vi "CANOpen_Initialize RT Driver.vi"(8 "error in (no error)":errorcluster, 11 "Device Reference in":T24 format="%.0x") -> (0 "error out":errorcluster, 3 "Configuration Cluster":T10={"Driver Settings"={"CANOpen Bus Settings"={"CANOpen Interface Name"=0, "Baud Rate"=0, "Termination"=FALSE, "Sync Period (ms)"=10, "Enable 9881"=FALSE, "RIO Device"=0, "Enable SYNC"=FALSE, "Scan & Print"=FALSE}, "Nodes"=[], "Node Ids"=[]}, "Data References"={"Hardware Input"={"FIFO"=refnum, "Channel Pairs"={"Chan Refs"=[], "Prev. Values"=[]}}, "Hardware Output"={"FIFO"=refnum, "Channel Pairs"={"Block Refs"=[], "Prev. Values"=[]}}}, "Bus Commands"={"Hardware Output"={"FIFO"=refnum, "Channel Pairs"={"Chan Refs"=[], "Prev. Values"=[]}}, "Hardware Input"={"FIFO"=refnum}}, "SDO Asynch"={"List SDO"={"FIFO Req"=refnum, "Req Chan."={"Chan Refs"=[], "NodeIndex"=[]}, "FIFO Resp"=refnum, "Resp Chan."={"Chan Refs"=[]}, "Node IDs"=[], "FIFO array"=[]}, "HW Dyn Write"={"FIFO Req"=refnum, "FIFO Resp"=refnum, "Req Chan."={"Chan Refs"=[], "Node IDs"=[]}, "Resp Chan."={"Chan Refs"=[]}}, "HW Dyn Read"={"FIFO Req"=refnum, "FIFO Resp"=refnum, "Req Chan."={"Chan Refs"=[], "Node IDs"=[]}, "Resp Chan."={"Chan Refs"=[]}}}, "Status NMT"={"Hardware Output"={"FIFO"=refnum, "Channel Pairs"={"Chan Refs"=[], "Prev. Values"=[], "Node index"=[]}}, "Hardware Input"={"FIFO"=refnum, "Channel Pairs"={"Chan Refs"=[], "Prev. Values"=[], "Node index"=[]}}}} {"Status NMT"."Hardware Output"."Channel Pairs"."Chan Refs"."Data Reference" format="%.0x"; "Status NMT"."Hardware Input"."Channel Pairs"."Chan Refs" format="%.0x"; "SDO Asynch"."HW Dyn Read"."Resp Chan."."Chan Refs" format="%.0x"; "SDO Asynch"."HW Dyn Read"."Req Chan."."Chan Refs" format="%.0x"; "SDO Asynch"."HW Dyn Write"."Resp Chan."."Chan Refs" format="%.0x"; "SDO Asynch"."HW Dyn Write"."Req Chan."."Chan Refs" format="%.0x"; "SDO Asynch"."List SDO"."Resp Chan."."Chan Refs" format="%.0x"; "SDO Asynch"."List SDO"."Req Chan."."Chan Refs" format="%.0x"; "Bus Commands"."Hardware Output"."Channel Pairs"."Chan Refs" format="%.0x"; "Data References"."Hardware Input"."Channel Pairs"."Chan Refs" format="%.0x"; "Data References"."Hardware Output"."Channel Pairs"."Block Refs"."Data Reference" format="%.0x"; "Driver Settings"."CANOpen Bus Settings"."Baud Rate" items=["1 Mbit/s"=0, "800 kbit/s"=1, "500 kbit/s"=2, "250 kbit/s"=3, "125 kbit/s"=4, "50 kbit/s"=6, "20 kbit/s"=7, "10 kbit/s"=8]; "Driver Settings"."CANOpen Bus Settings"."CANOpen Interface Name" items=["CANopen01", "CANopen02", "CANopen03", "CANopen04", "CANopen05", "CANopen06", "CANopen07", "CANopen08", "CANopen09", "CANopen10", "CANopen11", "CANopen12", "CANopen13", "CANopen14", "CANopen15", "CANopen16", "CANopen17", "CANopen18", "CANopen19", "CANopen20", "CANopen21", "CANopen22", "CANopen23", "CANopen24", "CANopen25", "CANopen26", "CANopen27", "CANopen28", "CANopen29", "CANopen30", "CANopen31", "CANopen32"]; "Driver Settings"."Nodes"."NMT"."Node init static SDO state" items=["start remote node"=1, "enter pre-operational"=128]; "Driver Settings"."Nodes"."NMT"."Node run state" items=["start remote node"=1, "stop remote node"=2, "enter pre-operational"=128, "reset node"=129, "reset communication"=130]; "Driver Settings"."Nodes"."Dynamic SDOs"."Block Data" format="%.0x"; "Driver Settings"."Nodes"."RPDOs"."PDO Channel" items=["PDO 1", "PDO 2", "PDO 3", "PDO 4"]; "Driver Settings"."Nodes"."TPDOs"."PDO Channel" items=["PDO 1", "PDO 2", "PDO 3", "PDO 4"]; "Driver Settings"."Nodes"."SDOs"."Block Data" format="%.0x"})   [LabVIEW 2013]
uses:
  <vilib>/NI Veristand/Custom Device API/Custom Device Item Ref.ctl
  CANOpen_Settings.ctl
  CANOpen_Node Settings.ctl
  Shared Code/CANOpen_Bus Settings.ctl
  Shared Code/CANOpen Interface Name.ctl
  <vilib>/CANopenLib/CANOPEN.llb/CANopen BaudRate.ctl
  CANOpen_Node Message Settings.ctl
  Shared Code/CANOpen_PDO Settings.ctl
  Shared Code/CANOpen_PDO Parameter Settings.ctl
  Shared Code/CANOpen_PDO Data Type.ctl
  System Explorer/SubVIs/CANopen Byte Order.ctl
  Shared Code/CANOpen_SDO Settings.ctl
  CANOpen_NMT Settings.ctl
  Async VIs/CANOpen_Main/SubVIs/CanOpen_NMT_Config.ctl
  Async VIs/CANOpen_Main/SubVIs/CanOpen_NMT_Static detect.ctl
  Async VIs/CANOpen_Main/SubVIs/CanOpen_Main Node Ids.ctl
  CANOpen_VS Data Refs.ctl
  <vilib>/NI Veristand/Custom Device API/Data Reference.ctl
  <vilib>/NI Veristand/Custom Device API/Block Data Reference.ctl
  CANOpen_VS Bidirectional Data Refs.ctl
  CANOpen_VS SDOs Data Refs.ctl
  Async VIs/CANOpen_Main/SubVIs/CanOpen_SDO Dynamic queue.ctl
  Shared Code/CANOpen_SDO queue W data.ctl
  Shared Code/CANOpen_SDO queue mode.ctl
  Shared Code/CANOpen_PDO Data Type in queue.ctl
  CANOpen_VS Status Management Data Refs.ctl
  Async VIs/CANOpen_Main/SubVIs/CanOpen_NMT_HWOut_ChannelPairs.ctl
  Async VIs/CANOpen_Main/SubVIs/CanOpen_NMT_HWIn_ChannelPairs.ctl
  CANOpen_xPDO VS Refs.ctl
  Shared Code/CANOpen_Get PDO Channel from Name.vi
  Shared Code/CANOpen_SetGet PDO Parameter Settings.vi
  CANOpen_SetGet NMT Settings.vi
  CANOpen_Initialize VS BiDirectional Data Refs.vi
  CANOpen_Search Channel Ref.vi
  CANOpen_Search Channel Refs.vi
  CANOpen_Initialize VS NMT Data Refs.vi
  <vilib>/NI Veristand/Custom Device Tools/Custom Device Utility Library/NI VeriStand - Search for All Items by GUID.vi
  <vilib>/NI Veristand/Custom Device API/Get Item Property (Variant).vi
  Shared Code/CANOpen Addon GUID Lookup Global.vi
  <vilib>/NI Veristand/Custom Device API/NI VeriStand - Get Item Children.vi
  <vilib>/NI Veristand/Custom Device Tools/Custom Device Utility Library/NI VeriStand - Search for Item by GUID.vi
  <vilib>/NI Veristand/Custom Device API/NI VeriStand - Get Channel Data Reference.vi
  <vilib>/NI Veristand/Custom Device API/NI VeriStand - Get Channel Block Data References.vi
  <vilib>/NI Veristand/Custom Device Tools/Custom Device Utility Library/Custom Device Utility Library.lvlib
  CANOpen Addon Custom Device.lvlib
  <vilib>/NI Veristand/Custom Device API/Custom Device API.lvlib
  Debug/SubVIs/Global debug.vi
panel:
  out "Array":T1[](array[typedef]) {"NMT"."Node init static SDO state" items=["start remote node"=1, "enter pre-operational"=128]; "NMT"."Node run state" items=["start remote node"=1, "stop remote node"=2, "enter pre-operational"=128, "reset node"=129, "reset communication"=130]; "Dynamic SDOs"."Block Data" format="%.0x"; "RPDOs"."PDO Channel" items=["PDO 1", "PDO 2", "PDO 3", "PDO 4"]; "RPDOs"."Parameters"."Bit Offset" max=8 step=1; "RPDOs"."Parameters"."Byte Offset" max=8 step=1; "TPDOs"."PDO Channel" items=["PDO 1", "PDO 2", "PDO 3", "PDO 4"]; "TPDOs"."Parameters"."Bit Offset" max=8 step=1; "TPDOs"."Parameters"."Byte Offset" max=8 step=1; "SDOs"."Block Data" format="%.0x"}
  # "LSB"
  # "MSB"
  # "LSB"
  # "MSB"
  # "LSB"
  # "MSB"
  # "LSB"
  # "MSB"
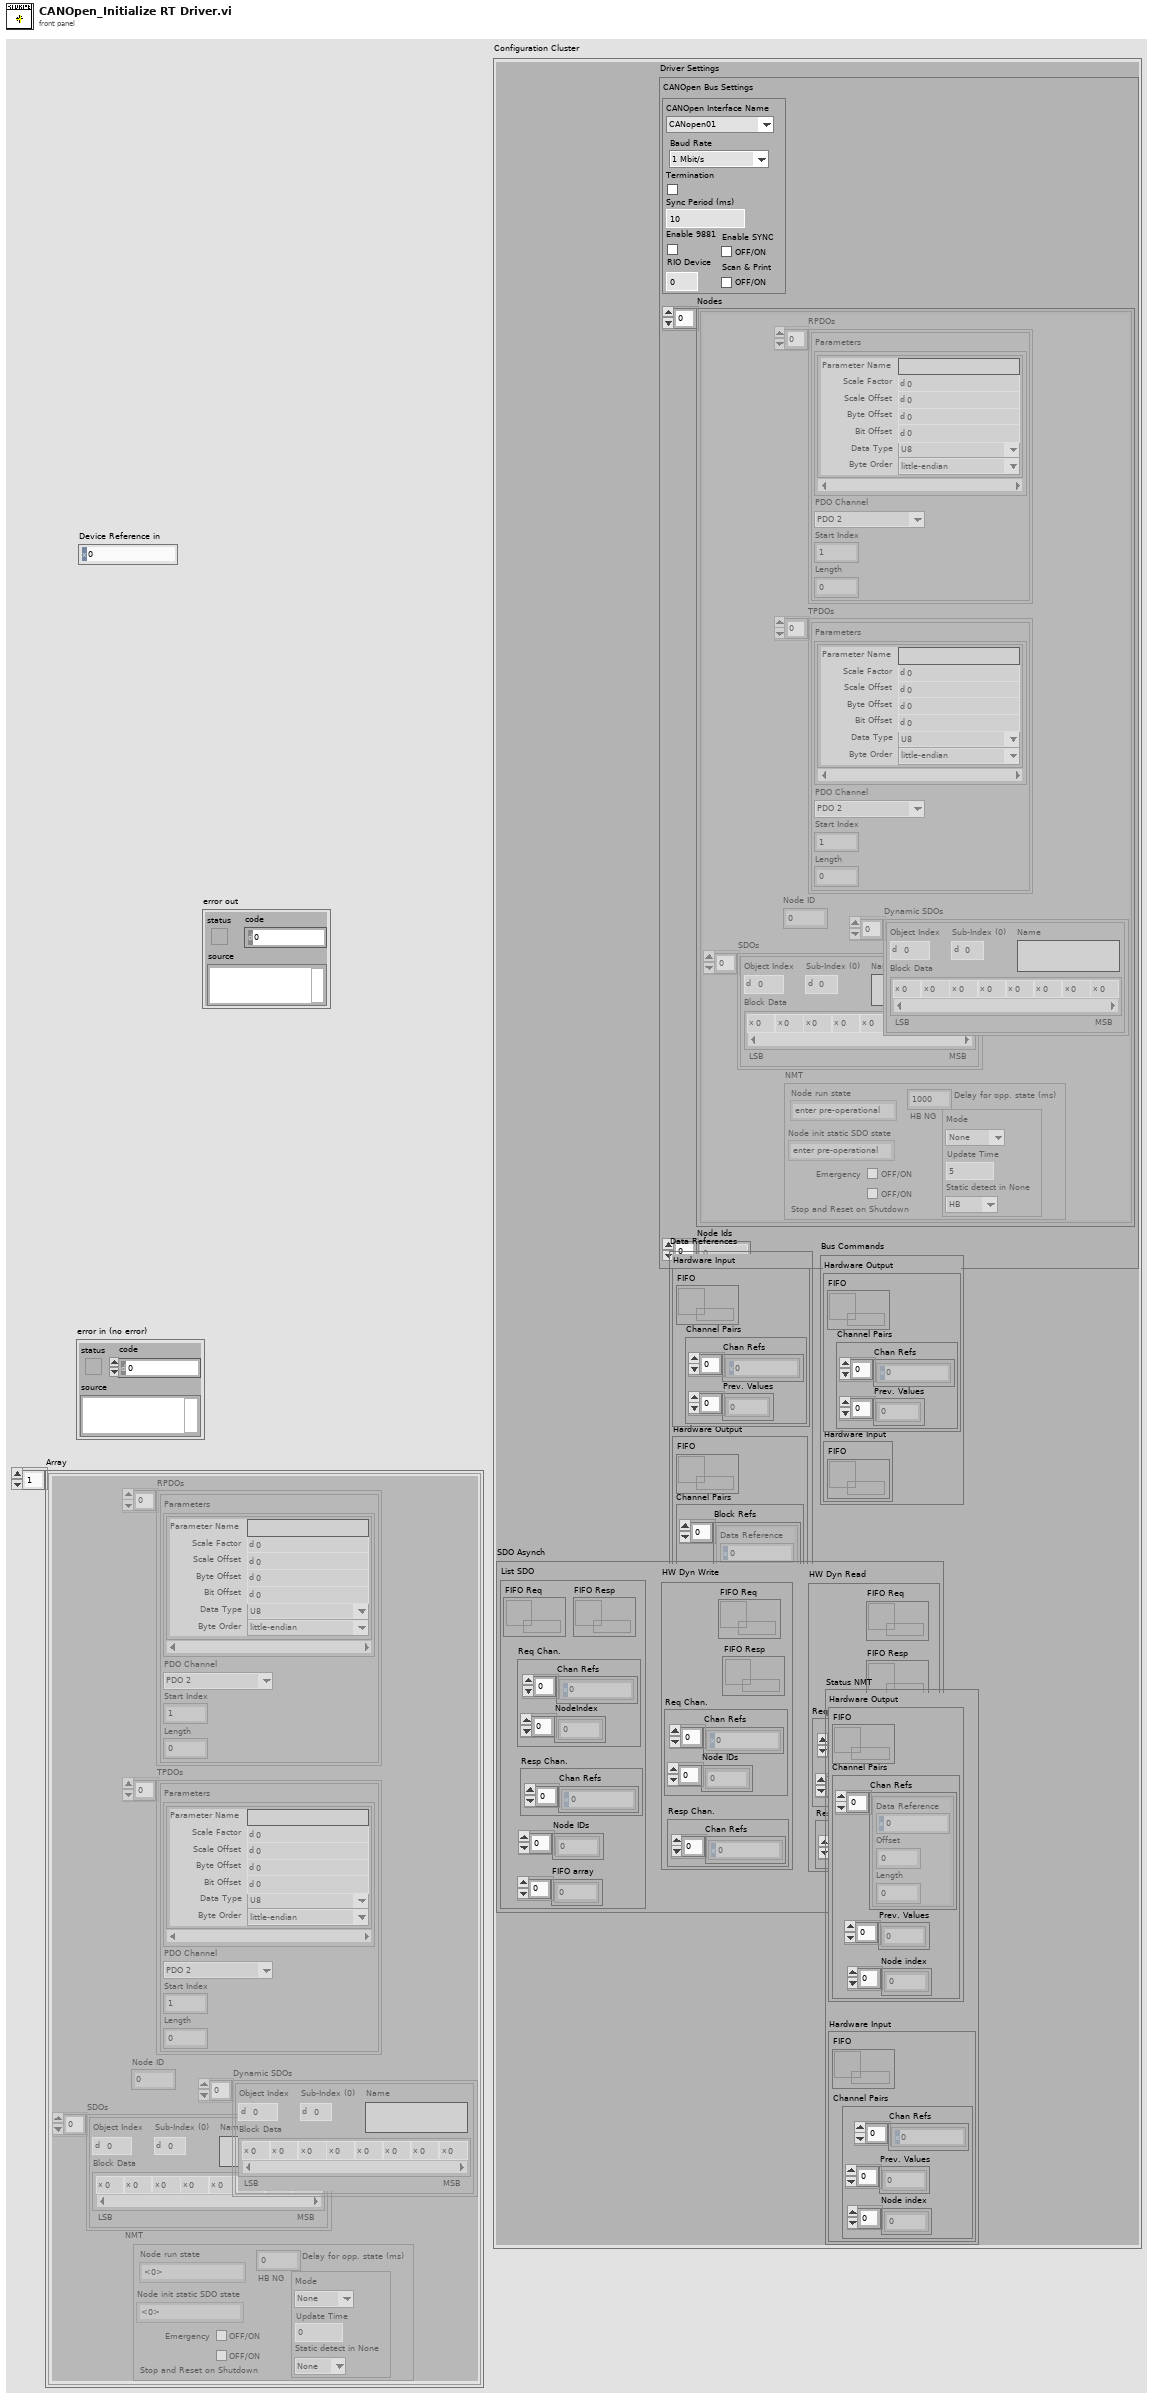
[diagram p1: front panel]
types:
  T1 = typedef "CANOpen_Node Message Settings.ctl" = cluster{"RPDOs":T2[], "TPDOs":T2[], "Node ID":u8, "SDOs":T6[], "Dynamic SDOs":T6[], "NMT":T7}
  T2 = typedef "CANOpen Addon Custom Device.lvlib/CANOpen_PDO Settings.ctl" = cluster{"Parameters":T3[], "PDO Channel":u8, "Start Index":u32, "Length":u32}
  T3 = typedef "CANOpen Addon Custom Device.lvlib/CANOpen_PDO Parameter Settings.ctl" = cluster{"Parameter Name":string, "Scale Factor":dbl, "Scale Offset":dbl, "Byte Offset":u8, "Bit Offset":u8, "Data Type":T4, "Byte Order":T5}
  T4 = typedef "CANOpen Addon Custom Device.lvlib/CANOpen_PDO Data Type.ctl" = enum16{"U8", "U16", "U32", "I8", "I16", "I32", "Single", "Double", "Boolean"}
  T5 = typedef "CANOpen Addon Custom Device.lvlib/CANopen Byte Order.ctl" = enum16{"big-endian network order", "little-endian"}
  T6 = typedef "CANOpen Addon Custom Device.lvlib/CANOpen_SDO Settings.ctl" = cluster{"Object Index":u16, "Sub-Index (0)":u8, "Block Data":u8[], "Name":string}
  T7 = typedef "CANOpen Addon Custom Device.lvlib/CANOpen_NMT Settings.ctl" = cluster{"Node run state":u16, "Emergency":bool, "HB NG":T8, "Delay for opp. state (ms)":dbl, "Node init static SDO state":u16, "Stop and Reset on Shutdown":bool}
  T8 = typedef "CANOpen Addon Custom Device.lvlib/CanOpen_NMT_Config.ctl" = cluster{"Mode":T9, "Update Time":u16, "Static detect in None":T9}
  T9 = typedef "CANOpen Addon Custom Device.lvlib/CanOpen_NMT_Static detect.ctl" = enum16{"None", "HB", "NG"}
  T10 = typedef "CANOpen_Settings.ctl" = cluster{"Driver Settings":T11, "Data References":T16, "Bus Commands":T19, "SDO Asynch":T20, "Status NMT":T21}
  T11 = typedef "CANOpen_Node Settings.ctl" = cluster{"CANOpen Bus Settings":T12, "Nodes":T1[], "Node Ids":T15}
  T12 = typedef "CANOpen Addon Custom Device.lvlib/CANOpen_Bus Settings.ctl" = cluster{"CANOpen Interface Name":T13, "Baud Rate":T14, "Termination":bool, "Sync Period (ms)":i64, "Enable 9881":bool, "RIO Device":u16, "Enable SYNC":bool, "Scan & Print":bool}
  T13 = typedef "CANOpen Addon Custom Device.lvlib/CANOpen Interface Name.ctl" = u32
  T14 = typedef "CANopen BaudRate.ctl" = u32
  T15 = typedef "CANOpen Addon Custom Device.lvlib/CanOpen_Main Node Ids.ctl" = u8[]
  T16 = typedef "CANOpen_VS Data Refs.ctl" = cluster{"Hardware Input":cluster{"FIFO":refnum<k33>, "Channel Pairs":cluster{"Chan Refs":T17[], "Prev. Values":dbl[]}}, "Hardware Output":cluster{"FIFO":refnum<k33>, "Channel Pairs":cluster{"Block Refs":T18[], "Prev. Values":dbl[]}}}
  T17 = typedef "Custom Device API.lvlib/Data Reference.ctl" = i32
  T18 = typedef "Custom Device API.lvlib/Block Data Reference.ctl" = cluster{"Data Reference":T17, "Offset":i32, "Length":i32}
  T19 = typedef "CANOpen_VS Bidirectional Data Refs.ctl" = cluster{"Hardware Output":cluster{"FIFO":refnum<k33>, "Channel Pairs":cluster{"Chan Refs":T17[], "Prev. Values":dbl[]}}, "Hardware Input":cluster{"FIFO":refnum<k33>}}
  T20 = typedef "CANOpen Addon Custom Device.lvlib/CANOpen_VS SDOs Data Refs.ctl" = cluster{"List SDO":cluster{"FIFO Req":refnum<k33>, "Req Chan.":cluster{"Chan Refs":T17[], "NodeIndex":dbl[]}, "FIFO Resp":refnum<k33>, "Resp Chan.":cluster{"Chan Refs":T17[]}, "Node IDs":u8[], "FIFO array":dbl[]}, "HW Dyn Write":cluster{"FIFO Req":refnum<k33>, "FIFO Resp":refnum<k33>, "Req Chan.":cluster{"Chan Refs":T17[], "Node IDs":u8[]}, "Resp Chan.":cluster{"Chan Refs":T17[]}}, "HW Dyn Read":cluster{"FIFO Req":refnum<k33>, "FIFO Resp":refnum<k33>, "Req Chan.":cluster{"Chan Refs":T17[], "Node IDs":u8[]}, "Resp Chan.":cluster{"Chan Refs":T17[]}}}
  T21 = typedef "CANOpen Addon Custom Device.lvlib/CANOpen_VS Status Management Data Refs.ctl" = cluster{"Hardware Output":cluster{"FIFO":refnum<k33>, "Channel Pairs":T22}, "Hardware Input":cluster{"FIFO":refnum<k33>, "Channel Pairs":T23}}
  T22 = typedef "CANOpen Addon Custom Device.lvlib/CanOpen_NMT_HWOut_ChannelPairs.ctl" = cluster{"Chan Refs":T18[], "Prev. Values":dbl[], "Node index":dbl[]}
  T23 = typedef "CANOpen Addon Custom Device.lvlib/CanOpen_NMT_HWIn_ChannelPairs.ctl" = cluster{"Chan Refs":T17[], "Prev. Values":dbl[], "Node index":dbl[]}
  T24 = typedef "Custom Device API.lvlib/Custom Device Item Ref.ctl" = u64
  T25 = typedef "CANOpen_xPDO VS Refs.ctl" = cluster{"Start Index":i32, "Child Refs":T24[]}
  T26 = typedef "Custom Device API.lvlib/Custom Device Item Info.ctl" = cluster{"Name":string, "Is Channel":bool, "GUID":string, "Is Waveform":bool}
  T27 = enum16{"open", "replace", "create", "open or create", "replace or create", "replace or create with confirmation"}
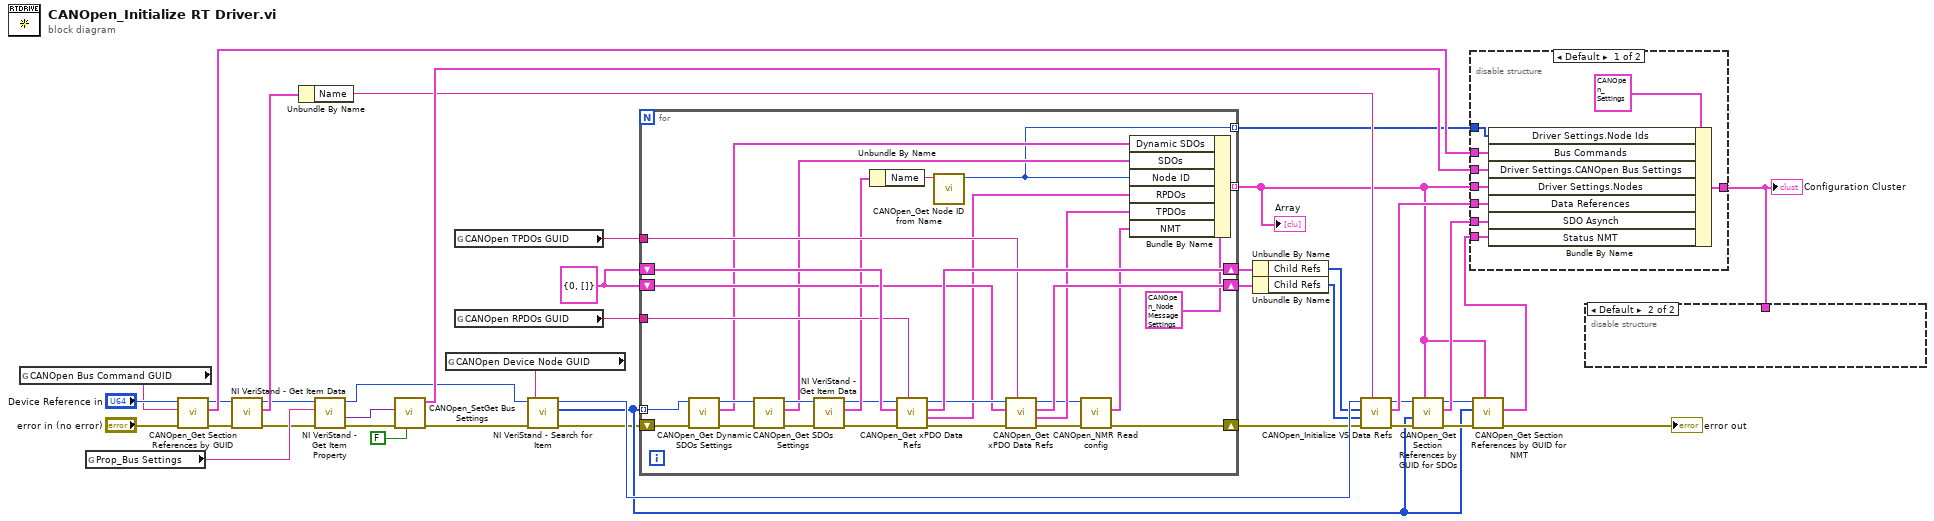
[diagram p0: block diagram]
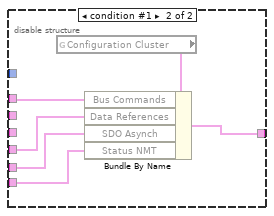
[diagram p2: hidden frame]
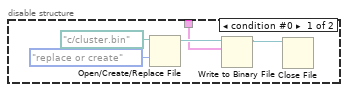
[diagram p3: hidden frame]
diagram:
  w18 = T25 {"Start Index"=0, "Child Refs"=[]} ("xPDOs")
  n1 = global read "CANOpen Addon GUID Lookup Global.vi" "CANOpen Bus Command GUID"() -> (w17:string)
  n2 = global read "CANOpen Addon GUID Lookup Global.vi" "Prop_Bus Settings"() -> (w31:string)
  n3 = call "CANOpen_Get Section References by GUID.vi"("error in (no error)"="error in (no error)", "Search GUID"=w17, "Device Ref"="Device Reference in") -> ("error out"=w12:errorcluster, "Data References"=w21:T19, "Device Ref out"=w13:T24)  [unwired: 6 in]
  n4 = call <vilib>:"NI VeriStand - Get Item Data.vi"("error in (no error)"=w12, "Item Ref in"=w13) -> ("error out"=w27:errorcluster, "Item Info"=w29:T26, "Item Ref out"=w28:T24)  [unwired: 6 in, 1 out]
  n5 = Unbundle By Name(w29) -> ("Name"=w26:string)
  n6 = call-poly <vilib>:"NI VeriStand - Get Item Property.vi"("error in (no error)"=w27, "Property Name"=w31, "Item Ref in"=w28) -> ("error out"=w33:errorcluster, "Value"=w34:variant, "Item Ref out"=w1:T24)  [unwired: 5 in, 1 out]
  n7 = call "CANOpen_SetGet Bus Settings.vi"("Set Parameters"=FALSE, "error in (no error)"=w33, "Parameters"=w34) -> ("error out"=w35:errorcluster, "CANOpen Bus Settings"=w30:T12)  [unwired: 6 in, 1 out]
  n8 = global read "CANOpen Addon GUID Lookup Global.vi" "CANOpen Device Node GUID"() -> (w36:string)
  n9 = global read "CANOpen Addon GUID Lookup Global.vi" "CANOpen TPDOs GUID"() -> (w38:string)
  n10 = global read "CANOpen Addon GUID Lookup Global.vi" "CANOpen RPDOs GUID"() -> (w37:string)
  n11 = call-poly <vilib>:"NI VeriStand - Search for Item.vi"("error in"=w35, "Item GUID"=w36, "Section Ref in"=w1) -> ("error out"=w2:errorcluster, "Item Refs"=w3:T24[], "Section Ref out"=w25:T24)  [unwired: 5 in, 1 out]
  n12 = for {
    tunnel: w3 -> [w47] mode=indexing
    tunnel: w37 -> [w67]
    shift-right: [w68] -> w40
    shift-left: w18 -> [w69]
    tunnel: w38 -> [w62]
    shift-right: [w63] -> w39
    shift-left: w18 -> [w64]
    shift-right: [w42] -> w16
    shift-left: w2 -> [w50]
    tunnel: [w55] -> w6 mode=indexing
    tunnel: [w45] -> w4 mode=indexing
    n13 = call "CANOpen_Get Dynamic SDOs Settings.vi"("error in"=w50, "Device Ref in"=w47) -> ("error out"=w49:errorcluster, "SDOs"=w46:T6[], "Device Ref out"=w48:T24)  [unwired: 7 in]
    n14 = call "CANOpen_Get SDOs Settings.vi"("error in"=w49, "Device Ref in"=w48) -> ("error out"=w52:errorcluster, "SDOs"=w51:T6[], "Device Ref out"=w53:T24)  [unwired: 7 in]
    n15 = call <vilib>:"NI VeriStand - Get Item Data.vi"("error in (no error)"=w52, "Item Ref in"=w53) -> ("error out"=w59:errorcluster, "Item Info"=w60:T26, "Item Ref out"=w54:T24)  [unwired: 6 in, 1 out]
    n16 = Unbundle By Name(w60) -> ("Name"=w61:string)
    n17 = call "CANOpen_Get xPDO Data Refs.vi"("xPDOs GUID"=w67, "error in (no error)"=w59, "State Variables"=w69, "Section Ref in"=w54) -> ("error out"=w66:errorcluster, "xPDOs"=w57:T2[], "xPDOs Out"=w68:T25, "Section Ref out"=w65:T24)  [unwired: 4 in]
    n18 = call "CANOpen_Get Node ID from Name.vi"("Node ID Name"=w61) -> ("Node ID"=w45:u8)  [unwired: 10 in]
    n19 = call "CANOpen_Get xPDO Data Refs.vi"("xPDOs GUID"=w62, "error in (no error)"=w66, "State Variables"=w64, "Section Ref in"=w65) -> ("error out"=w43:errorcluster, "xPDOs"=w56:T2[], "xPDOs Out"=w63:T25, "Section Ref out"=w44:T24)  [unwired: 4 in]
    n20 = call "CANOpen_NMR Read config.vi"("error in (no error)"=w43, "Section Ref in"=w44) -> ("error out"=w42:errorcluster, "NMT"=w41:T7)  [unwired: 7 in, 1 out]
    n21 = Bundle By Name(cluster=T1 {"RPDOs"=[], "TPDOs"=[], "Node ID"=0, "SDOs"=[], "Dynamic SDOs"=[], "NMT"={"Node run state"=0, "Emergency"=FALSE, "HB NG"={"Mode"=enum."None", "Update Time"=0, "Static detect in None"=enum."None"}, "Delay for opp. state (ms)"=0.0, "Node init static SDO state"=0, "Stop and Reset on Shutdown"=FALSE}}, "Dynamic SDOs"=w46, "SDOs"=w51, "Node ID"=w45, "RPDOs"=w57, "TPDOs"=w56, "NMT"=w41) -> (w55:T1)
  }
  "Array" <- w6
  n22 = Unbundle By Name(w40) -> ("Child Refs"=w19:T24[])
  n23 = Unbundle By Name(w39) -> ("Child Refs"=w20:T24[])
  n24 = call "CANOpen_Initialize VS Data Refs.vi"("Name"=w26, "error in (no error)"=w16, "Hardware Input Refs"=w20, "Hardware Output Refs"=w19, "Device Ref"=w25) -> ("error out"=w14:errorcluster, "Data References"=w24:T16, "Device Ref out"=w15:T24)  [unwired: 4 in]
  n25 = call "CANOpen_Get Section References by GUID for SDOs.vi"("Nodes"=w6, "error in (no error)"=w14, "Node Refs"=w3, "Device Ref"=w15) -> ("error out"=w8:errorcluster, "Data References"=w11:T20, "Device Ref out"=w9:T24)  [unwired: 5 in]
  n26 = call "CANOpen_Get Section References by GUID for NMT.vi"("Nodes"=w6, "error in (no error)"=w8, "Node Refs"=w3, "Device Ref"=w9) -> ("error out"=→"error out":errorcluster, "Data References"=w5:T21)  [unwired: 5 in, 1 out]
  n27 = disable-structure shown="Default" {
    disable-tunnel: w30 -> [w77 _]
    disable-tunnel: w24 -> [w76 w81]
    disable-tunnel: w21 -> [w75 w82]
    disable-tunnel: w11 -> [w74 w80]
    disable-tunnel: w6 -> [w73 _]
    disable-tunnel: [w72 w83] -> w10
    disable-tunnel: w5 -> [w71 w79]
    disable-tunnel: w4 -> [w70 _]
    frame condition #0 (active) {
      n28 = Bundle By Name(cluster=T10 {"Driver Settings"={"CANOpen Bus Settings"={"CANOpen Interface Name"=0, "Baud Rate"=0, "Termination"=FALSE, "Sync Period (ms)"=0, "Enable 9881"=FALSE, "RIO Device"=0, "Enable SYNC"=FALSE, "Scan & Print"=FALSE}, "Nodes"=[], "Node Ids"=[]}, "Data References"={"Hardware Input"={"FIFO"=refnum, "Channel Pairs"={"Chan Refs"=[], "Prev. Values"=[]}}, "Hardware Output"={"FIFO"=refnum, "Channel Pairs"={"Block Refs"=[], "Prev. Values"=[]}}}, "Bus Commands"={"Hardware Output"={"FIFO"=refnum, "Channel Pairs"={"Chan Refs"=[], "Prev. Values"=[]}}, "Hardware Input"={"FIFO"=refnum}}, "SDO Asynch"={"List SDO"={"FIFO Req"=refnum, "Req Chan."={"Chan Refs"=[], "NodeIndex"=[]}, "FIFO Resp"=refnum, "Resp Chan."={"Chan Refs"=[]}, "Node IDs"=[], "FIFO array"=[]}, "HW Dyn Write"={"FIFO Req"=refnum, "FIFO Resp"=refnum, "Req Chan."={"Chan Refs"=[], "Node IDs"=[]}, "Resp Chan."={"Chan Refs"=[]}}, "HW Dyn Read"={"FIFO Req"=refnum, "FIFO Resp"=refnum, "Req Chan."={"Chan Refs"=[], "Node IDs"=[]}, "Resp Chan."={"Chan Refs"=[]}}}, "Status NMT"={"Hardware Output"={"FIFO"=refnum, "Channel Pairs"={"Chan Refs"=[], "Prev. Values"=[], "Node index"=[]}}, "Hardware Input"={"FIFO"=refnum, "Channel Pairs"={"Chan Refs"=[], "Prev. Values"=[], "Node index"=[]}}}} ("Configuration Cluster"), "Driver Settings.Node Ids"=w70, "Bus Commands"=w75, "Driver Settings.CANOpen Bus Settings"=w77, "Driver Settings.Nodes"=w73, "Data References"=w76, "SDO Asynch"=w74, "Status NMT"=w71) -> (w72:T10)
    }
    frame condition #1 {
      n29 = global read "Global debug.vi" "Configuration Cluster"() -> (w84:T10)
      n30 = Bundle By Name(cluster=w84, "Bus Commands"=w82, "Data References"=w81, "SDO Asynch"=w80, "Status NMT"=w79) -> (w83:T10)
    }
  }
  "Configuration Cluster" <- w10
  n31 = disable-structure shown="Default" {
    disable-tunnel: w10 -> [w85 _]
    frame condition #0 {
      n32 = Open/Create/Replace File(file path (use dialog)=path "c:/cluster.bin", operation (0:open)=T27."replace or create") -> (refnum out=w89:refnum<file>)  [unwired: 4 in, 2 out]
      n33 = Write to Binary File(file (use dialog)=w89, data=w85) -> (refnum out=w86:refnum<file>)  [unwired: 4 in, 2 out]
      n34 = Close File(refnum=w86) -> ()  [unwired: 1 in, 2 out]
    }
    frame condition #1 (active) {
    }
  }
